vi "get waveform - voltage range scaled.vi"(8 "error in (no error)":errorcluster caption="에러 입력(에러 없음)", 11 "Text File 입력":refnum<class "Text File.lvclass">) -> (0 "error out":errorcluster caption="에러 출력", 2 "scaled waveform":waveform(dbl), 3 "Text File 출력":refnum<class "Text File.lvclass">)   [LabVIEW 2020, in "Text File.lvclass"]
uses:
  Text File.lvclass
  Waveform Obj/Waveform Obj.lvclass/Waveform Obj.ctl
  Waveform Obj/Accessors/Read voltage range.vi
  Text File.lvclass/Text File.ctl
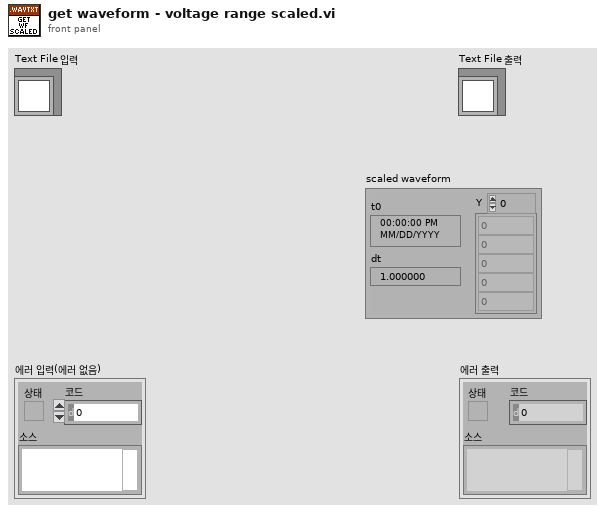
[diagram p1: front panel]
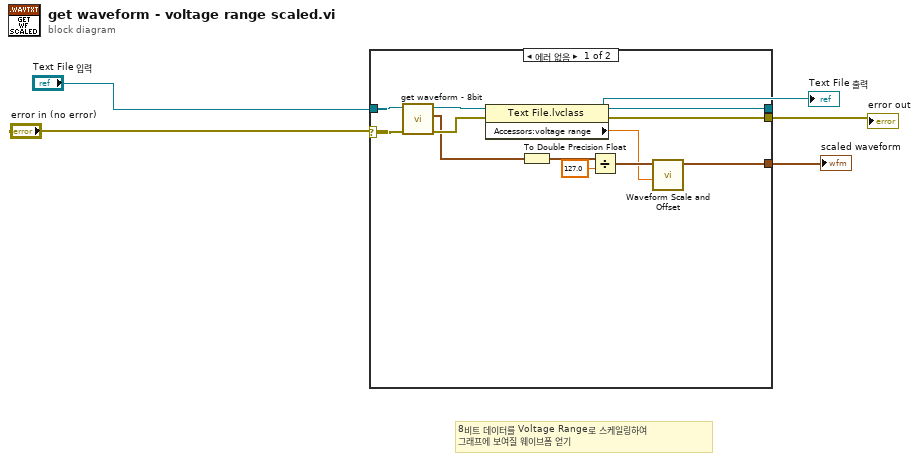
[diagram p0: block diagram]
diagram:
  # "8비트 데이터를 Voltage Range로 스케일링하여\n그래프에 보여질 웨이브폼 얻기"
  n1 = case shown="에러 없음" "error in (no error)" {
    selector: "error in (no error)" -> [w17 w19]
    tunnel: [w12 w19] -> w5
    tunnel: [w11 w18] -> w3
    tunnel: "Text File 입력" -> [w8 w18]
    tunnel: [w13 _] -> w4
    frame No Error {
      n2 = call-dynamic "get waveform - 8bit.vi"("error in (no error)"=w17, "Text File 입력"=w8) -> ("error out"=w9:errorcluster, "8bit waveform"=w6:waveform(i8), "Text File 출력"=w7:refnum<class "Text File.lvclass">)  [unwired: 6 in, 1 out]
      n3 = property class="Text File.lvclass"(reference=w7, error in=w9) -> (reference out=w11:refnum<class "Text File.lvclass">, error out=w12:errorcluster, "Accessors:voltage range"=w10:dbl)
      n4 = To Double Precision Float(number=w6) -> (double precision float=w16:waveform(dbl))
      n5 = Divide(x=w16, y=127.0) -> (x/y=w14:waveform(dbl))
      n6 = call <vilib>:"Waveform Scale and Offset.vi"("scale"=w10, "waveform in"=w14) -> ("waveform out"=w13:waveform(dbl))  [unwired: 8 in, 1 out]
    }
    frame Error {
    }
  }
  "error out" <- w5
  "Text File 출력" <- w3
  "scaled waveform" <- w4
